vi "Init Hardware.vi"(8 "error in (no error)":errorcluster, 11 "Application in":refnum<class "Application.lvclass">) -> (0 "error out":errorcluster, 3 "Application out":refnum<class "Application.lvclass">)   [LabVIEW 2018, in "Application.lvlib" / "Application.lvclass"]
uses:
  Application.lvclass
  C:/Program Files/National Instruments/LabVIEW 2018/vi.lib/ActorFramework/Actor/Actor.lvclass
  Hardware/Tiff Writer/Tiff Writer/Tiff Writer.lvclass
  Application.lvclass/Application.ctl
  <vilib>/ActorFramework/Actor/Actor.lvclass
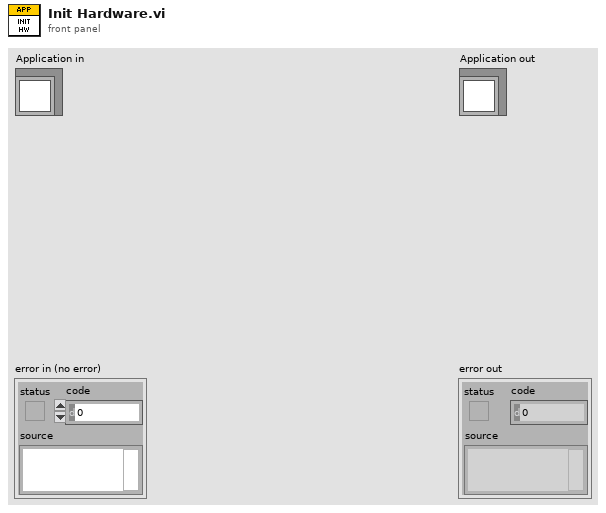
[diagram p1: front panel]
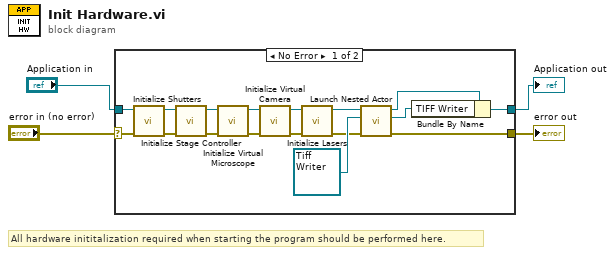
[diagram p0: block diagram]
diagram:
  # "All hardware inititalization required when starting the program should be performed here."
  n1 = case shown="No Error" "error in (no error)" {
    selector: "error in (no error)" -> [w21 w23]
    tunnel: [w10 w23] -> w3
    tunnel: [w7 w22] -> w1
    tunnel: "Application in" -> [w12 w22]
    frame No Error {
      n2 = call-dynamic "Initialize Shutters.vi"("error in (no error)"=w21, "Application in"=w12) -> ("error out"=w20:errorcluster, "Application out"=w18:refnum<class "Application.lvclass">)  [unwired: 8 in]
      n3 = call-dynamic "Initialize Stage Controller.vi"("error in (no error)"=w20, "Application in"=w18) -> ("error out"=w19:errorcluster, "Application out"=w17:refnum<class "Application.lvclass">)  [unwired: 8 in]
      n4 = call-dynamic "Initialize Virtual Microscope.vi"("error in (no error)"=w19, "Application in"=w17) -> ("error out"=w15:errorcluster, "Application out"=w16:refnum<class "Application.lvclass">)  [unwired: 8 in]
      n5 = call-dynamic "Initialize Virtual Camera.vi"("error in (no error)"=w15, "Application in"=w16) -> ("error out"=w13:errorcluster, "Application out"=w14:refnum<class "Application.lvclass">)  [unwired: 8 in]
      n6 = call-dynamic "Initialize Lasers.vi"("error in (no error)"=w13, "Application in"=w14) -> ("error out"=w8:errorcluster, "Application out"=w9:refnum<class "Application.lvclass">)  [unwired: 8 in]
      n7 = call <vilib>:"Launch Nested Actor.vi"("error in (no error)"=w8, "Nested Actor"=refnum<class "Tiff Writer.lvclass"> refnum ("Tiff Writer.lvlib:Tiff Writer.lvclass"), "Caller Actor in"=w9) -> ("error out"=w10:errorcluster, "Nested Actor's Enqueuer"=w5:refnum<class "Message Enqueuer.lvclass">, "Caller Actor out"=w6:refnum<class "Application.lvclass">)  [unwired: 6 in]
      n8 = Bundle By Name(cluster=w6, "TIFF Writer"=w5) -> (w7:refnum<class "Application.lvclass">)
    }
    frame Error {
    }
  }
  "error out" <- w3
  "Application out" <- w1
